vi "testChem1.vi"() -> ()   [LabVIEW 2012]
uses:
  <userlib>/ImageProcessing/InitCamera_NTSC.vi
  <userlib>/ImageProcessing/FilterGreenPlane.vi
  <userlib>/ImageProcessing/FilterRedPlane.vi
panel:
  out "appended array":i32[][](array[numeric])
  out "Centroid 4":cluster{"X":dbl, "Y":dbl}
  out "Centroid 3":cluster{"X":dbl, "Y":dbl}
  out "Centroid 2":cluster{"X":dbl, "Y":dbl}
  out "Centroid":cluster{"X":dbl, "Y":dbl}
  out "initialized array 2":dbl[][](array[numeric])
  out "Intensity Graph":u32[][](graph)
  out "image":picture
  in  "Stop":bool
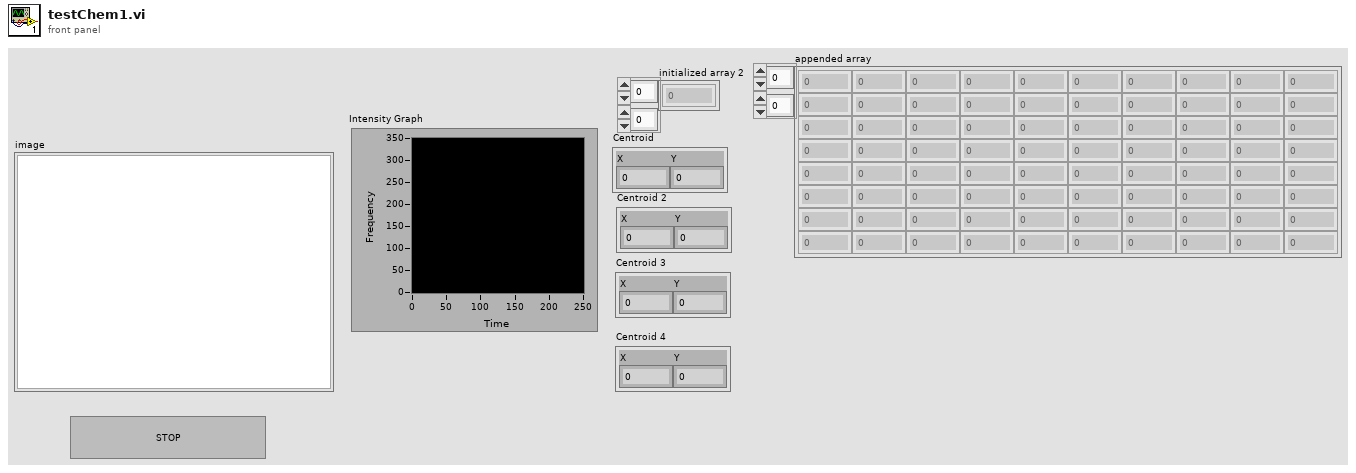
[diagram p1: front panel]
types:
  T1 = typedef "QT_Ref.ctl" = refnum<k1>
  T2 = cluster{"Width":u16, "Style":enum32{"Solid", "Dash", "Dot", "DashDot", "DashDotDot"}}
  T3 = typedef "QT_Image.ctl" = cluster{"Width":i32, "Height":i32, "Depth":i32, "data":u8[], "Compressed data":u8[], "Color table":u32[], "Duration":i32, "Options":i32, "Timestamp":i32, "ID":i32, "Reserved":i32, "Dialogs":u32}
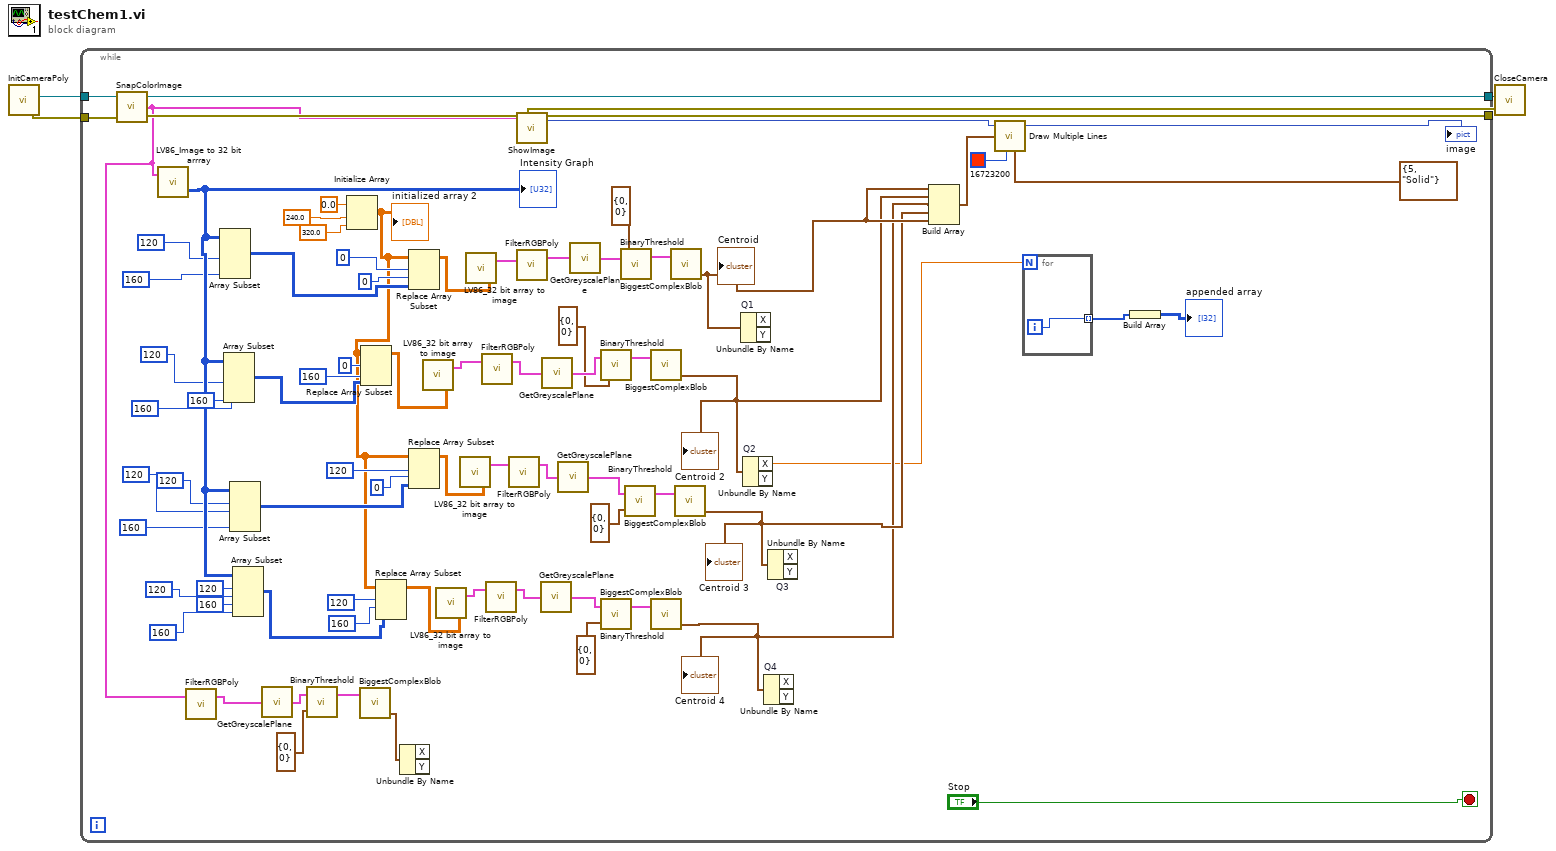
[diagram p0: block diagram]
diagram:
  n1 = call-poly <userlib>:"InitCameraPoly.vi"() -> ("error out"=w1:errorcluster, "QT Ref Out"=w2:T1)  [unwired: 2 in]
  n2 = while {
    tunnel: w1 -> [w80]
    tunnel: w2 -> [w79]
    tunnel: [w78] -> w3
    tunnel: [w77] -> w4
    stop <- "Stop" stop-if-true
    n3 = call <userlib>:"SnapColorImage.vi"("error in (no error)"=w80, "QT Ref In"=w79) -> ("error out"=w78:errorcluster, "Image Out"=w13:T3, "QT Ref Out"=w77:T1)  [unwired: 1 in]
    n4 = call <userlib>:"LV86_Image to 32 bit arrray.vi"("Image In"=w13) -> ("Intensity Graph"=w75:u32[][])  [unwired: 1 in, 1 out]
    "Intensity Graph" <- w75
    n5 = call-poly <userlib>:"FilterRGBPoly.vi"("Image in"=w13) -> ("Image out"=w9:T3)  [unwired: 1 in, 1 out]
    n6 = Array Subset(array=w75, length (row)=120 ("length"), length (col)=160 ("length")) -> (w51:u32[][])  [unwired: 2 in]
    n7 = Array Subset(array=w75, length (row)=120 ("length"), index (col)=160 ("index"), length (col)=160 ("length")) -> (w62:u32[][])  [unwired: 1 in]
    n8 = Array Subset(array=w75, index (row)=120 ("index"), length (row)=120 ("length"), length (col)=160 ("length")) -> (w45:u32[][])  [unwired: 1 in]
    n9 = Array Subset(array=w75, index (row)=120 ("index"), length (row)=120 ("length"), index (col)=160 ("index"), length (col)=160 ("length")) -> (w42:u32[][])
    n10 = call <userlib>:"GetGreyscalePlane.vi"("Image In"=w9) -> ("Greyscale  Out"=w8:T3)
    n11 = call <userlib>:"BinaryThreshold.vi"("threshold"=cluster{u8, u8} {0, 0}, "Image In"=w8) -> ("Image Out"=w7:T3)  [unwired: 1 in]
    n12 = Initialize Array(0.0 ("element"), 240.0 ("element"), 320.0 ("element")) -> (w41:dbl[][])
    "initialized array 2" <- w41
    n13 = call <userlib>:"BiggestComplexBlob.vi"("Image in"=w7) -> ("Centroid"=w5:cluster{"X":dbl, "Y":dbl})  [unwired: 1 in, 2 out]
    n14 = Replace Array Subset(array=w41, new element=w62, index (row)=0, index (col)=160 ("index (row)")) -> (w61:dbl[][])
    n15 = Replace Array Subset(array=w41, new element=w42, index (row)=120, index (col)=160 ("index (row)")) -> (w39:dbl[][])
    n16 = Unbundle By Name(w5) -> ()  [unwired: 2 out]
    n17 = Replace Array Subset(array=w41, new element=w51, index (row)=0, index (col)=0 ("index (row)")) -> (w50:dbl[][])
    n18 = Replace Array Subset(array=w41, new element=w45, index (row)=120, index (col)=0 ("index (row)")) -> (w40:dbl[][])
    n19 = call <userlib>:"LV86_32 bit array to image.vi"("Intensity Graph"=w61) -> ("Image Out"=w38:T3)  [unwired: 2 in]
    n20 = call <userlib>:"LV86_32 bit array to image.vi"("Intensity Graph"=w39) -> ("Image Out"=w36:T3)  [unwired: 2 in]
    n21 = call <userlib>:"LV86_32 bit array to image.vi"("Intensity Graph"=w40) -> ("Image Out"=w37:T3)  [unwired: 2 in]
    n22 = call <userlib>:"LV86_32 bit array to image.vi"("Intensity Graph"=w50) -> ("Image Out"=w49:T3)  [unwired: 2 in]
    n23 = call-poly <userlib>:"FilterRGBPoly.vi"("Image in"=w38) -> ("Image out"=w35:T3)  [unwired: 1 in, 1 out]
    n24 = call-poly <userlib>:"FilterRGBPoly.vi"("Image in"=w36) -> ("Image out"=w33:T3)  [unwired: 1 in, 1 out]
    n25 = call-poly <userlib>:"FilterRGBPoly.vi"("Image in"=w37) -> ("Image out"=w34:T3)  [unwired: 1 in, 1 out]
    n26 = call <userlib>:"ShowImage.vi"("Image"=w13) -> ("image"=w26:picture)  [unwired: 2 in, 1 out]
    n27 = call-poly <userlib>:"FilterRGBPoly.vi"("Image in"=w49) -> ("Image out"=w48:T3)  [unwired: 1 in, 1 out]
    n28 = call <userlib>:"GetGreyscalePlane.vi"("Image In"=w33) -> ("Greyscale  Out"=w27:T3)
    n29 = call <userlib>:"GetGreyscalePlane.vi"("Image In"=w35) -> ("Greyscale  Out"=w29:T3)
    n30 = call <userlib>:"GetGreyscalePlane.vi"("Image In"=w34) -> ("Greyscale  Out"=w28:T3)
    n31 = call <userlib>:"GetGreyscalePlane.vi"("Image In"=w48) -> ("Greyscale  Out"=w47:T3)
    n32 = call <userlib>:"BinaryThreshold.vi"("threshold"=cluster{u8, u8} {0, 0}, "Image In"=w29) -> ("Image Out"=w32:T3)  [unwired: 1 in]
    n33 = call <userlib>:"BinaryThreshold.vi"("threshold"=cluster{u8, u8} {0, 0}, "Image In"=w27) -> ("Image Out"=w30:T3)  [unwired: 1 in]
    n34 = call <userlib>:"BinaryThreshold.vi"("threshold"=cluster{u8, u8} {0, 0}, "Image In"=w47) -> ("Image Out"=w46:T3)  [unwired: 1 in]
    n35 = call <userlib>:"BinaryThreshold.vi"("threshold"=cluster{u8, u8} {0, 0}, "Image In"=w28) -> ("Image Out"=w31:T3)  [unwired: 1 in]
    n36 = call <userlib>:"BiggestComplexBlob.vi"("Image in"=w32) -> ("Centroid"=w16:cluster{"X":dbl, "Y":dbl})  [unwired: 1 in, 2 out]
    "Centroid 2" <- w16
    n37 = call <userlib>:"BiggestComplexBlob.vi"("Image in"=w30) -> ("Centroid"=w14:cluster{"X":dbl, "Y":dbl})  [unwired: 1 in, 2 out]
    "Centroid 4" <- w14
    n38 = call <userlib>:"BiggestComplexBlob.vi"("Image in"=w46) -> ("Centroid"=w17:cluster{"X":dbl, "Y":dbl})  [unwired: 1 in, 2 out]
    "Centroid" <- w17
    n39 = call <userlib>:"BiggestComplexBlob.vi"("Image in"=w31) -> ("Centroid"=w15:cluster{"X":dbl, "Y":dbl})  [unwired: 1 in, 2 out]
    "Centroid 3" <- w15
    n40 = Unbundle By Name "Q1"(w17) -> ()  [unwired: 2 out]
    n41 = Unbundle By Name "Q2"(w16) -> ("X"=w12:dbl)  [unwired: 1 out]
    n42 = Unbundle By Name "Q4"(w14) -> ()  [unwired: 2 out]
    n43 = Unbundle By Name "Q3"(w15) -> ()  [unwired: 2 out]
    n44 = Build Array(w17, w16, w14, w15, w17) -> (w24:cluster{"X":dbl, "Y":dbl}[])
    n45 = call <vilib>:"Draw Multiple Lines.vi"("picture"=w26, "line endpoints"=w24, "color(black)"=u32 16723200, "pen"=T2 {"Width"=5, "Style"=enum."Solid"}) -> ("new picture"=→"image":picture)  [unwired: 5 in]
    n46 = for {
      N: w12 -> [_]
      tunnel: [w81] -> w10 mode=indexing
      i -> [w81]
    }
    n47 = Build Array(w10) -> (→"appended array":i32[][])
  }
  n48 = call <userlib>:"CloseCamera.vi"("error in (no error)"=w3, "QT Ref In"=w4) -> ()  [unwired: 1 in, 1 out]
